vi "OP500Z8P_Conti_BT3564.vi"(8 "errin":errorcluster, 10 "chemin de base":path, 11 "VISAin":refnum<visa-resource-name>) -> (0 "errout":errorcluster, 3 "R mOhm":dbl)   [LabVIEW 2020]
uses:
  <instrlib>/HIOKI BT356X Series/Public/_Initialize/Initialize_serial.vi
  <instrlib>/HIOKI BT356X Series/Public/Action-Status/_Trigger/Init cont.vi
  <instrlib>/HIOKI BT356X Series/Public/Configure/_Trigger/Trigger.vi
  <instrlib>/HIOKI BT356X Series/Public/Configure/_Range/Voltage range.vi
  <instrlib>/HIOKI BT356X Series/Public/Configure/_Range/Resistance range.vi
  <instrlib>/HIOKI BT356X Series/HIOKI BT356X Series.lvlib
panel:
  out "Output Str":string[](array[string])
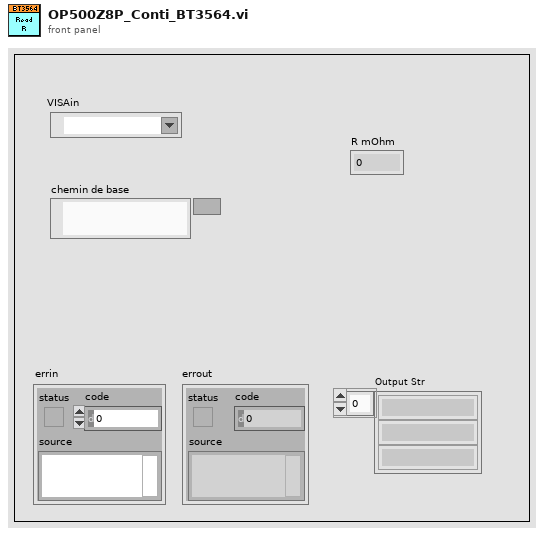
[diagram p1: front panel]
types:
  T1 = enum32{"BT3561A", "BT3562A", "BT3563A", "BT3562", "BT3563", "BT3564", "3561"}
  T2 = cluster{"Timeout":dbl, "Baud":u32, "Vmin":dbl, "Vmax":dbl, "RminMili":dbl, "Rmaxmili":dbl, "Vrange":dbl}
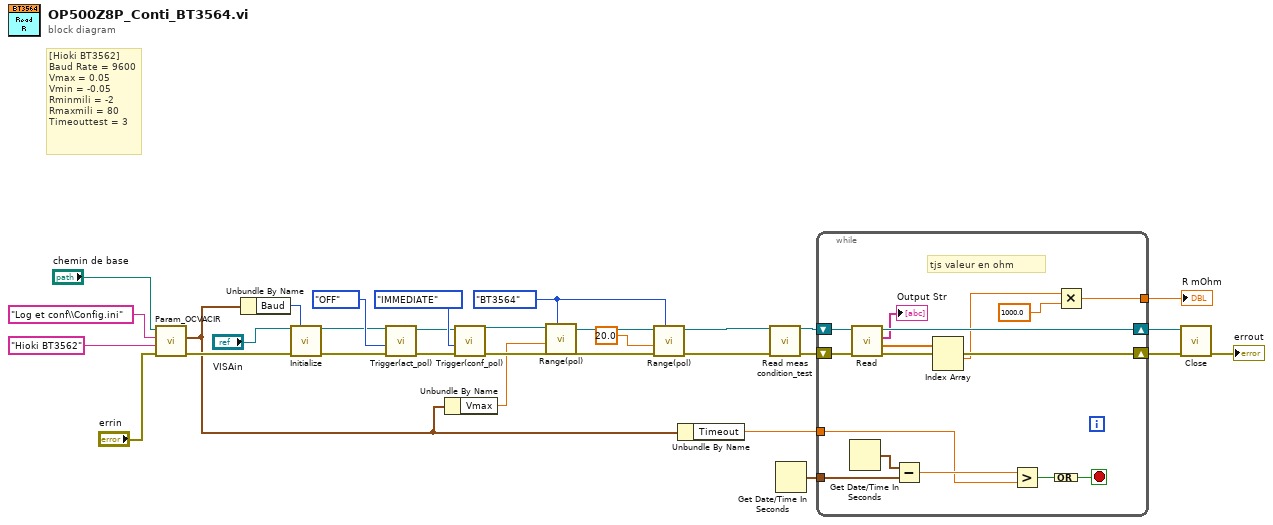
[diagram p0: block diagram]
diagram:
  w8 = T1."BT3564" ("Model")
  # "[Hioki BT3562]\nBaud Rate = 9600\nVmax = 0.05\nVmin = -0.05\nRminmili = -2\nRmaxmili = 80\nTimeouttest = 3"
  n1 = call "Param_OCVACIR.vi"("errin"="errin", "section"="Hioki BT3562", "Chaîne"="Log et conf\\Config.ini", "pathin"="chemin de base") -> ("Errout"=w17:errorcluster, "DATA"=w4:T2)  [unwired: 6 in]
  n2 = Unbundle By Name(w4) -> ("Baud"=w15:u32)
  n3 = call-poly <instrlib>:"Initialize.vi"("VISA resource name"="VISAin", "Baud Rate"=w15, "error in (no error)"=w17) -> ("VISA resource name out"=w24:refnum<visa-resource-name>, "error out"=w23:errorcluster)  [unwired: 11 in]
  n4 = call-poly <instrlib>:"Trigger(act_pol).vi"("error in (no error)"=w23, "Do not idle set"=enum16{"ON", "OFF"}."OFF", "VISA session"=w24) -> ("error out"=w27:errorcluster, "dup VISA session"=w26:refnum<visa-resource-name>)  [unwired: 6 in, 1 out]
  n5 = Unbundle By Name(w4) -> ("Vmax"=w3:dbl)
  n6 = call-poly <instrlib>:"Trigger(conf_pol).vi"("error in (no error)"=w27, "Trigger set"=enum16{"IMMEDIATE", "EXTERNAL"}."IMMEDIATE", "VISA session"=w26) -> ("error out"=w11:errorcluster, "dup VISA session"=w12:refnum<visa-resource-name>)  [unwired: 6 in, 1 out]
  n7 = call-poly <instrlib>:"Range(pol).vi"("Model"=w8, "error in (no error)"=w11, "Voltage Range set"=w3, "VISA session"=w12) -> ("error out"=w9:errorcluster, "dup VISA session"=w10:refnum<visa-resource-name>)  [unwired: 5 in, 1 out]
  n8 = call-poly <instrlib>:"Range(pol).vi"("Model"=w8, "error in (no error)"=w9, "Resistance range set"=20.0, "VISA session"=w10) -> ("error out"=w6:errorcluster, "dup VISA session"=w5:refnum<visa-resource-name>)  [unwired: 5 in, 1 out]
  n9 = Unbundle By Name(w4) -> ("Timeout"=w14:dbl)
  n10 = call <instrlib>:"Read meas condition_test.vi"("VISA RefnumIn"=w5, "ErrIn"=w6) -> ("VISA Refnumo"=w21:refnum<visa-resource-name>, "Errout"=w22:errorcluster)  [unwired: 9 in, 3 out]
  n11 = Get Date/Time In Seconds() -> (seconds since 1Jan1904=w20:timestamp)
  n12 = while {
    shift-right: [w43] -> w31
    shift-left: w21 -> [w44]
    shift-right: [w42] -> w30
    shift-left: w22 -> [w45]
    tunnel: w20 -> [w40]
    tunnel: w14 -> [w37]
    tunnel: [w32] -> w2
    stop <- w35 stop-if-true
    # "tjs valeur en ohm"
    n13 = Get Date/Time In Seconds() -> (seconds since 1Jan1904=w41:timestamp)
    n14 = call <instrlib>:"Read.vi"("error in (no error)"=w45, "VISA session"=w44) -> ("error out"=w42:errorcluster, "Output Val"=w46:dbl[], "Output Str"=→"Output Str":string[], "dup VISA session"=w43:refnum<visa-resource-name>)  [unwired: 6 in]
    n15 = Subtract(x=w41, y=w40) -> (x-y=w39:dbl)
    n16 = Index Array(array=w46) -> (element #1=w34:dbl)  [unwired: 2 in, 1 out]
    n17 = Greater?(x=w39, y=w37) -> (0:w38:bool)
    n18 = Compound Arithmetic op=OR ("Opérateur arithmétique")(w38) -> (w35:bool)
    n19 = Multiply(x=w34, y=1000.0) -> (x*y=w32:dbl)
  }
  "R mOhm" <- w2
  n20 = call <instrlib>:"Close.vi"("error in (no error)"=w30, "VISA resource name"=w31) -> ("error out"=→"errout":errorcluster)  [unwired: 9 in]
